vi "ResistanceMatrix.vi"() -> ()   [LabVIEW 2014]
panel:
  out "String 4":string
  out "Array 3":dbl[][](array[numeric]) format="%#_2g"
  out "String":string
  out "Array 2":string[](array[string])
  out "String 6":string
  in  "error in (no error)":errorcluster
  out "error out":errorcluster
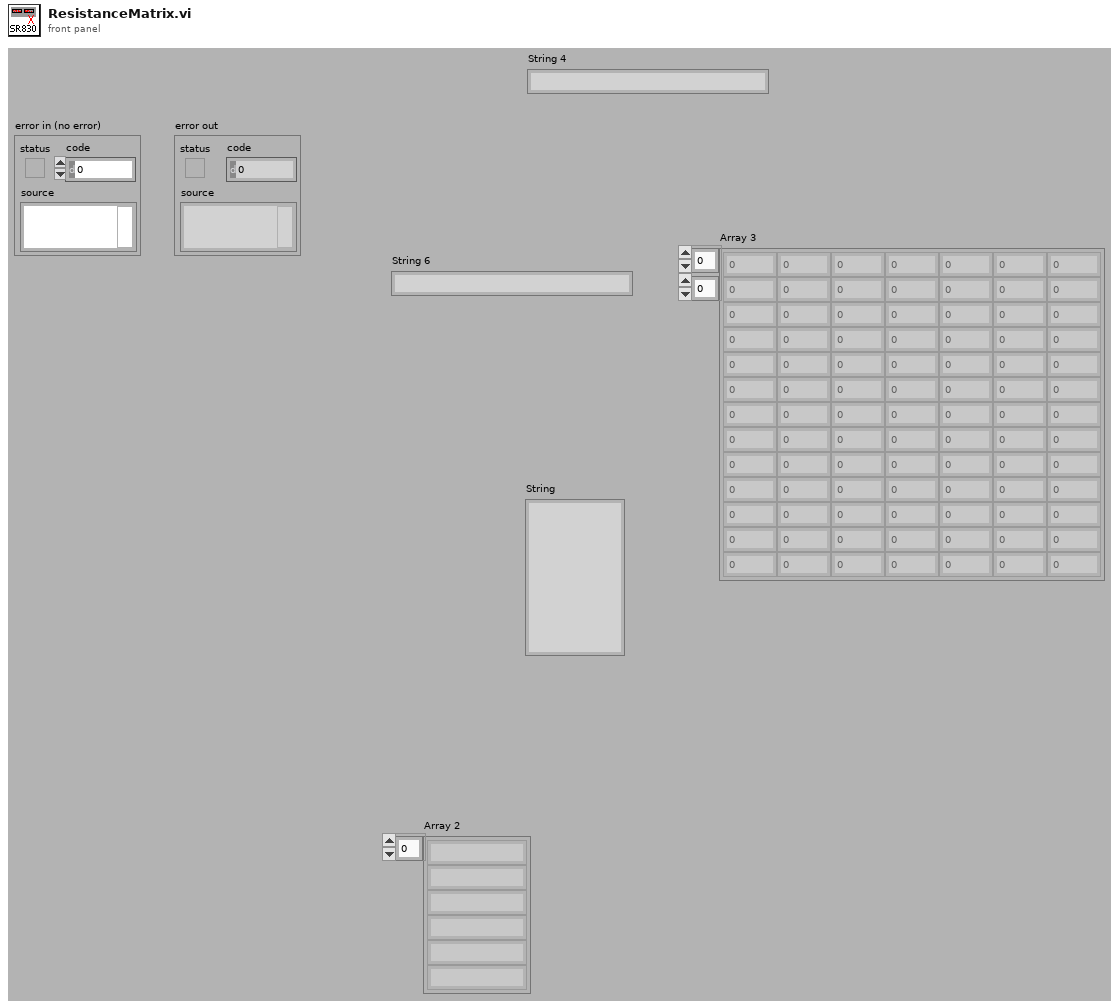
[diagram p1: front panel]
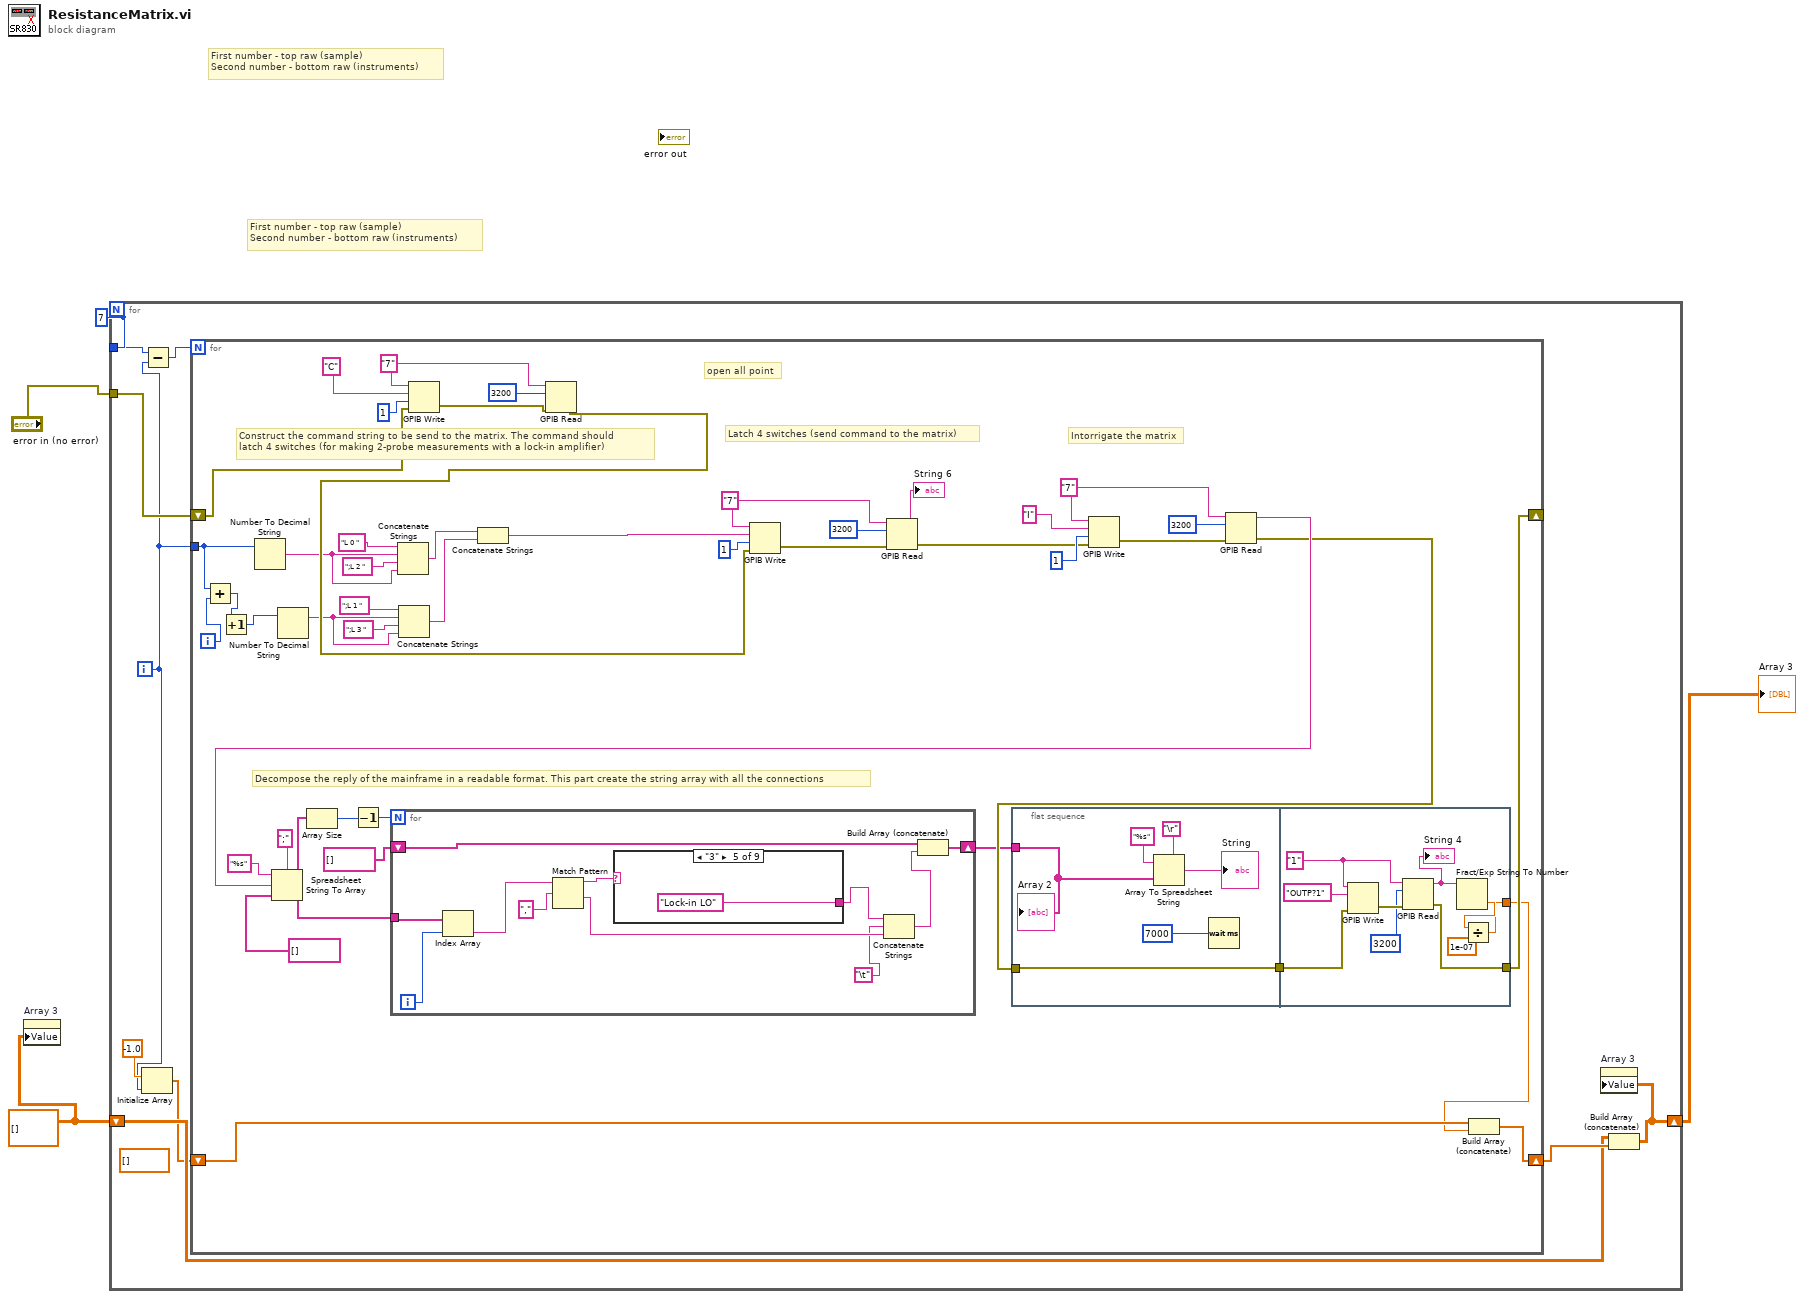
[diagram p0: block diagram]
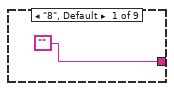
[diagram p2: hidden frame]
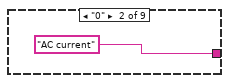
[diagram p3: hidden frame]
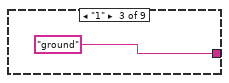
[diagram p4: hidden frame]
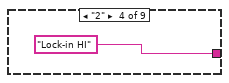
[diagram p5: hidden frame]
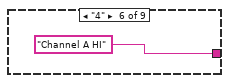
[diagram p6: hidden frame]
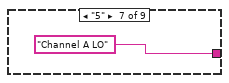
[diagram p7: hidden frame]
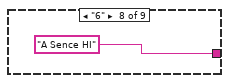
[diagram p8: hidden frame]
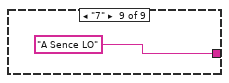
[diagram p9: hidden frame]
diagram:
  w1 = sgl[][] []
  w4 = 7
  # "First number - top raw (sample)\nSecond number - bottom raw (instruments)"
  # "First number - top raw (sample)\nSecond number - bottom raw (instruments)"
  n1 = property on="Array 3" class="Arr (strict)"("Value"=w1) -> ()  [unwired: 2 in, 2 out]
  n2 = for {
    N: w4 -> [_]
    tunnel: "error in (no error)" -> [w13]
    tunnel: w4 -> [w12]
    shift-right: [w8] -> w2
    shift-left: w1 -> [w9]
    i -> [w6]
    (unwired) sgl[] []
    n3 = Initialize Array(sgl -1.0, w6) -> (w5:sgl[])
    n4 = Subtract(x=w12, y=w6) -> (x-y=w11:i32)
    n5 = for {
      N: w11 -> [_]
      tunnel: w6 -> [w20]
      shift-right: [w33] -> _
      shift-left: w13 -> [w27]
      shift-right: [w16] -> w10
      shift-left: w5 -> [w17]
      i -> [w19]
      w29 = "7"
      w46 = "7"
      w57 = "7"
      # "open all point"
      # "Decompose the reply of the mainframe in a readable format. This part create the string array with all the connections"
      # "Intorrigate the matrix"
      # "Latch 4 switches (send command to the matrix)"
      # "Construct the command string to be send to the matrix. The command should\nlatch 4 switches (for making 2-probe measurements with a lock-in amplifier)"
      n6 = Add(x=w20, y=w19) -> (x+y=w18:i32)
      n7 = Increment(x=w18) -> (x+1=w50:i32)
      n8 = Number To Decimal String(number=w20) -> (decimal integer string=w25:string)  [unwired: 1 in]
      n9 = Number To Decimal String(number=w50) -> (decimal integer string=w24:string)  [unwired: 1 in]
      n10 = Concatenate Strings("L 0 ", w25, ";L 2 ", w25) -> (w22:string)
      n11 = Concatenate Strings(";L 1 ", w24, ";L 3 ", w24) -> (w21:string)
      n12 = GPIB Write(0:w29, 1:"C", 2:1, 3:w27) -> (6:w32:errorcluster)  [unwired: 1 in, 1 out]
      n13 = Concatenate Strings(w22, w21) -> (w23:string)
      n14 = GPIB Read(0:w29, 1:3200, 3:w32) -> (7:w26:errorcluster)  [unwired: 2 in, 2 out]
      n15 = GPIB Write(0:w57, 1:w23, 2:1, 3:w26) -> (6:w59:errorcluster)  [unwired: 1 in, 1 out]
      n16 = GPIB Read(0:w57, 1:3200, 3:w59) -> (5:→"String 6":string, 7:w36:errorcluster)  [unwired: 2 in, 1 out]
      n17 = flat-sequence {
        tunnel: w35 -> [w84]
        tunnel: w34 -> [w83]
        tunnel: [w84] -> w15
        tunnel: [w90] -> w33
        tunnel: w15 -> [w91]
        tunnel: [w86] -> w14
        frame #0 {
          n18 = Array To Spreadsheet String(delimiter (Tab)="\r", array=w83, 3:"%s") -> (spreadsheet string=→"String":string)
          n19 = Wait (ms)(milliseconds to wait=7000) -> ()  [unwired: 1 out]
          "Array 2" <- w83
        }
        frame #1 {
          w94 = "1"
          n20 = GPIB Write(0:w94, 1:"OUTP?1", 3:w91) -> (6:w95:errorcluster)  [unwired: 2 in, 1 out]
          n21 = GPIB Read(0:w94, 1:3200, 3:w95) -> (5:w89:string, 7:w90:errorcluster)  [unwired: 2 in, 1 out]
          "String 4" <- w89
          n22 = Fract/Exp String To Number(string=w89) -> (number=w88:dbl)  [unwired: 3 in, 1 out]
          n23 = Divide(x=w88, y=1e-07) -> (x/y=w86:dbl)
        }
      }
      n24 = GPIB Write(0:w46, 1:"I", 2:1, 3:w36) -> (6:w49:errorcluster)  [unwired: 1 in, 1 out]
      n25 = GPIB Read(0:w46, 1:3200, 3:w49) -> (5:w44:string, 7:w35:errorcluster)  [unwired: 2 in, 1 out]
      n26 = Spreadsheet String To Array(delimiter (Tab)=";", format string="%s", spreadsheet string=w44, array type (2D Dbl)=string[] []) -> (array=w41:string[])
      n27 = Array Size(array=w41) -> (size(s)=w40:i32)
      n28 = Decrement(x=w40) -> (x-1=w39:i32)
      n29 = for {
        N: w39 -> [_]
        tunnel: w41 -> [w70]
        shift-right: [w64] -> w34
        shift-left: string[] [] -> [w65]
        i -> [w69]
        n30 = Index Array(array=w70, index=w69) -> (element=w67:string)
        n31 = Match Pattern(string=w67, regular expression=",") -> (before substring=w63:string, after substring=w61:string)  [unwired: 1 in, 2 out]
        n32 = case shown="\"3\"" w63 {
          tunnel: ["" "AC current" "ground" "Lock-in HI" "Lock-in LO" "Channel A HI" "Channel A LO" "A Sence HI" "A Sence LO"] -> w62
          frame "8", Default {
          }
          frame "0" {
          }
          frame "1" {
          }
          frame "2" {
          }
          frame "3" {
          }
          frame "4" {
          }
          frame "5" {
          }
          frame "6" {
          }
          frame "7" {
          }
        }
        n33 = Concatenate Strings(w62, "\t", w61) -> (w66:string)
        n34 = Build Array (concatenate)(w65, w66) -> (w64:string[])
      }
      n35 = Build Array (concatenate)(w17, w14) -> (w16:dbl[])
    }
    n36 = Build Array (concatenate)(w9, w10) -> (w8:dbl[][])
    n37 = property on="Array 3" class="Arr (strict)"("Value"=w8) -> ()  [unwired: 2 in, 2 out]
  }
  "Array 3" <- w2
